vi "sendNoAckToClient.vi"(8 "error in (no error)":errorcluster, 9 "cmdLost":bool, 10 "tcpPacket":T1, 11 "tcpServer in":refnum<class "TcpServer.lvclass">) -> (0 "error out":errorcluster, 3 "tcpServer out":refnum<class "TcpServer.lvclass">)   [LabVIEW 2018, in "TcpServer.lvclass"]
doc: "Send the noAck to the TCP Client."
uses:
  TcpServer.lvclass
  typedef/tcpPacketTypeDef.ctl
panel:
  out "tcpPacket":T1
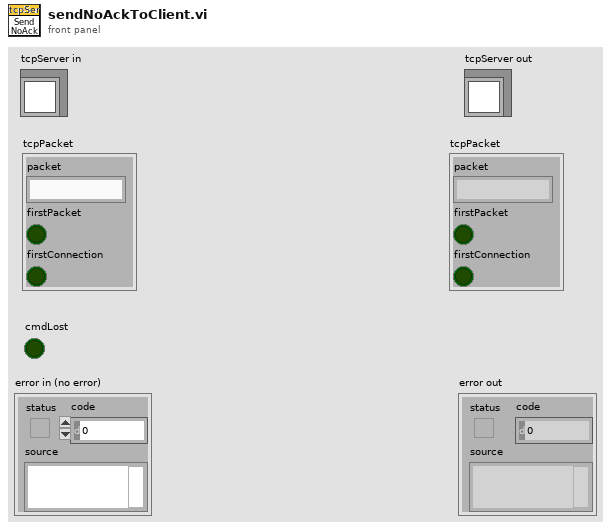
[diagram p1: front panel]
types:
  T1 = typedef "TcpServer.lvclass/tcpPacketTypeDef.ctl" = cluster{"packet":string, "firstPacket":bool, "firstConnection":bool}
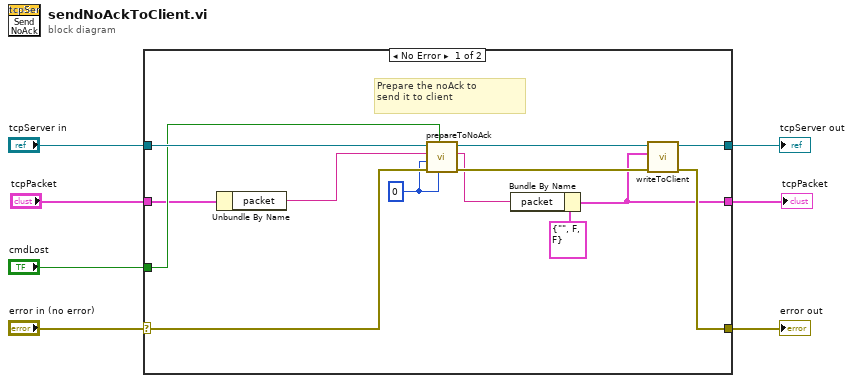
[diagram p0: block diagram]
diagram:
  n1 = case shown="No Error" "error in (no error)" {
    selector: "error in (no error)" -> [w16 w23]
    tunnel: [w19 w23] -> w6
    tunnel: [w20 w22] -> w4
    tunnel: "tcpServer in" -> [w18 w22]
    tunnel: [w11 w21] -> w1
    tunnel: "cmdLost" -> [w10 _]
    tunnel: "tcpPacket" -> [w9 w21]
    frame No Error {
      w12 = 0 ("lostCmdId")
      # "Prepare the noAck to\nsend it to client"
      n2 = Unbundle By Name(w9) -> ("packet"=w14:string)
      n3 = call "prepareToNoAck.vi"("iteration"=w12, "cmdLost"=w10, "error in (no error)"=w16, "lostCmdId"=w12, "cmd"=w14, "TcpServer in"=w18) -> ("error out"=w15:errorcluster, "JSON string"=w13:string, "TcpServer out"=w17:refnum<class "TcpServer.lvclass">)  [unwired: 3 in]
      n4 = Bundle By Name(cluster=T1 {"packet"="", "firstPacket"=FALSE, "firstConnection"=FALSE} ("tcpPacket"), "packet"=w13) -> (w11:T1)
      n5 = call "writeToClient.vi"("error in (no error)"=w15, "packetConnID"=w11, "tcpServer in"=w17) -> ("error out"=w19:errorcluster, "tcpServer out"=w20:refnum<class "TcpServer.lvclass">)  [unwired: 7 in]
    }
    frame Error {
    }
  }
  "error out" <- w6
  "tcpServer out" <- w4
  "tcpPacket" <- w1
